vi "Draw ByRef.vi"(8 "error in (no error)":errorcluster, 11 "ShapeRef":refnum<data-value>) -> (0 "error out":errorcluster, 2 "Raw Image":string, 3 "ShapeRef 2":refnum<data-value>)   [LabVIEW 2017, in "LV Image Editor Framework.lvlib" / "Shape.lvclass"]
uses:
  Shape.lvclass
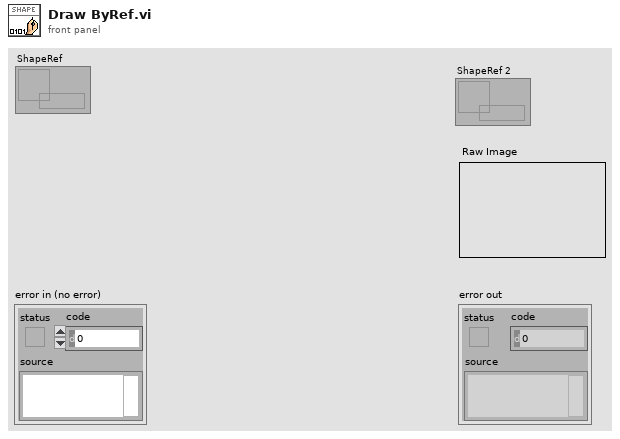
[diagram p1: front panel]
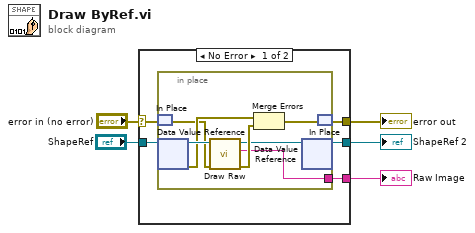
[diagram p0: block diagram]
diagram:
  n1 = case shown="No Error" "error in (no error)" {
    selector: "error in (no error)" -> [w8 w19]
    tunnel: [w7 w19] -> w4
    tunnel: "ShapeRef" -> [w10 w18]
    tunnel: [w9 w18] -> w2
    tunnel: [w6 _] -> w1
    frame No Error {
      n2 = in-place {
        in-place-border: [w12] -> w6
        n3 = in-place-match #1(w8) -> (w14:errorcluster)
        n4 = in-place-dvr #2(w10) -> (w17:refnum<class "Shape.lvclass">, w16:errorcluster)
        n5 = call "Draw Raw.vi"("error in (no error)"=w14, "Shape in"=w17) -> ("error out"=w15:errorcluster, "Raw"=w12:string, "Shape out"=w11:refnum<class "Shape.lvclass">)  [unwired: 7 in]
        n6 = Merge Errors(w16, w15) -> (w13:errorcluster)
        n7 = in-place-dvr #2(w11) -> (w9:refnum<data-value>)  [unwired: 1 out]
        n8 = in-place-match #1(w13) -> (w7:errorcluster)
      }
    }
    frame Error {
    }
  }
  "error out" <- w4
  "ShapeRef 2" <- w2
  "Raw Image" <- w1
